vi "test_Basic RTcRIO Deployment.vi"(8 "error in (no error)":errorcluster, 11 "TestCase in":refnum<class "TLCD System Tests.lvclass">) -> (0 "error out":errorcluster, 3 "TestCase out":refnum<class "TLCD System Tests.lvclass">)   [LabVIEW 2019, in "TLCD System Tests.lvclass"]
uses:
  TLCD System Tests.lvclass
  C:/Users/nitest/Desktop/NI VS Custom Device Testing Tools/VeriStandTestCase/VeriStandTestCase.lvclass
  NI VS Custom Device Testing Tools/VeriStandTestUtilities/TargetPlatform.ctl
  NI VS Custom Device Testing Tools/VeriStandTestUtilities/SystemDefinitionInformation.ctl
  NI VS Custom Device Testing Tools/VeriStandTestUtilities/TargetInformation.ctl
  NI VS Custom Device Testing Tools/VeriStandTestUtilities/ChassisInformation.ctl
  <vilib>/addons/_JKI Toolkits/VI Tester/TestCase.llb/TestCase.lvclass
  TLCD Test Class/TLCD Test Class.lvclass
  C:/Program Files (x86)/National Instruments/LabVIEW 2019/vi.lib/addons/_JKI Toolkits/VI Tester/TestCase.llb/TestCase.lvclass
  NI VS Custom Device Testing Tools/VeriStandTestUtilities/VeriStandTestUtilities.lvlib
panel:
  out "System Definition Information":T1
  out "Active Configuration":T4
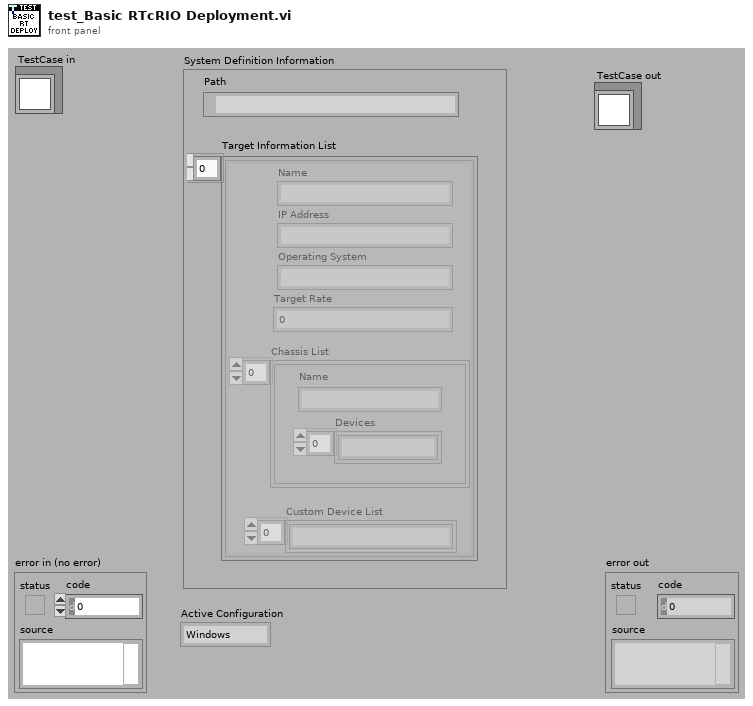
[diagram p1: front panel]
types:
  T1 = typedef "VeriStandTestUtilities.lvlib/SystemDefinitionInformation.ctl" = cluster{"Path":path, "Target Information List":T2[]}
  T2 = typedef "VeriStandTestUtilities.lvlib/TargetInformation.ctl" = cluster{"Name":string, "IP Address":string, "Operating System":string, "Target Rate":dbl, "Chassis List":T3[], "Custom Device List":string[]}
  T3 = typedef "VeriStandTestUtilities.lvlib/ChassisInformation.ctl" = cluster{"Name":string, "Devices":string[]}
  T4 = typedef "VeriStandTestUtilities.lvlib/TargetPlatform.ctl" = enum16{"Windows", "Linux64CRIO", "Linux64PXI", "LinuxARM", "PharLap"}
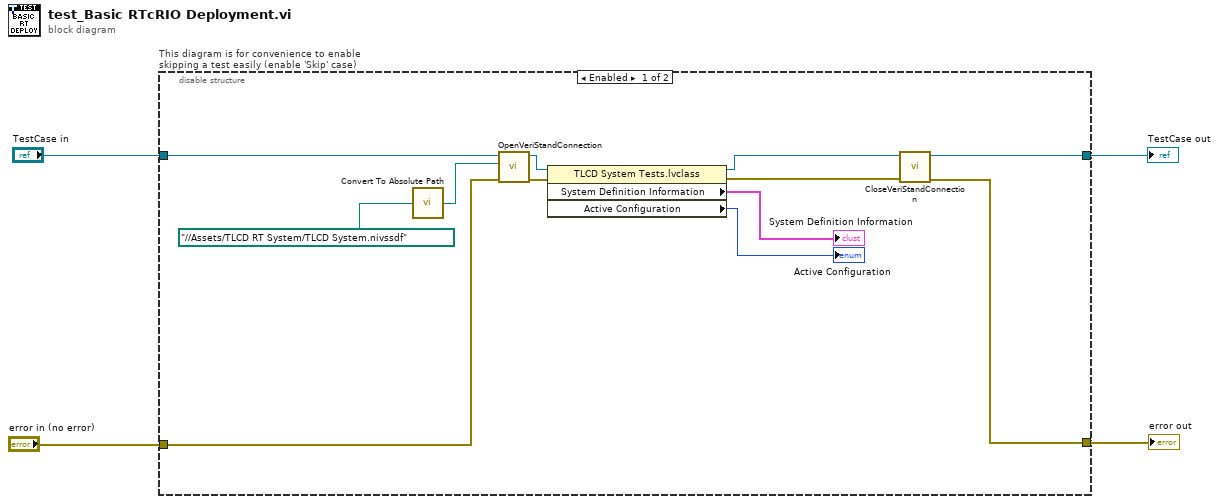
[diagram p0: block diagram]
diagram:
  n1 = disable-structure "This diagram is for convenience to enable skipping a test easily (enable 'Skip' case)" shown="Enabled" {
    disable-tunnel: "TestCase in" -> [w14 w20]
    disable-tunnel: [w11 w18] -> w1
    disable-tunnel: [w12 w19] -> w3
    disable-tunnel: "error in (no error)" -> [w15 w17]
    frame Enabled {
      n2 = call "Convert To Absolute Path.vi"("System Definition File Path"=path "../../Assets/TLCD RT System/TLCD System.nivssdf" ("relative base path")) -> ("Absolute path"=w13:path)
      n3 = call-dynamic "OpenVeriStandConnection.vi"("error in (no error)"=w15, "System Definition File"=w13, "VeriStand Test Case in"=w14) -> ("error out"=w10:errorcluster, "VeriStand Test Case out"=w9:refnum<class "TLCD System Tests.lvclass">)  [unwired: 6 in, 1 out]
      n4 = property class="TLCD System Tests.lvclass"(reference=w9, error in=w10) -> (reference out=w8:refnum<class "TLCD System Tests.lvclass">, error out=w7:errorcluster, "System Definition Information"=→"System Definition Information":T1, "Active Configuration"=→"Active Configuration":T4)
      n5 = call-dynamic "CloseVeriStandConnection.vi"("error in (no error)"=w7, "VeriStand Test Case in"=w8) -> ("error out"=w12:errorcluster, "VeriStand Test Case out"=w11:refnum<class "TLCD System Tests.lvclass">)  [unwired: 8 in]
    }
    frame Disabled {
      # "skip test result while test is under development"
      n6 = call <vilib>:"skip.vi"("error in (no error)"=w17, "TestCase in"=w20) -> ("error out"=w19:errorcluster, "TestCase out"=w18:refnum<class "TLCD System Tests.lvclass">)  [unwired: 8 in]
    }
  }
  "error out" <- w3
  "TestCase out" <- w1
